vi "SpectrumCursor_getCenter.vi"(5 "Value":cluster{dbl[], dbl[]}) -> (0 "cursor2X":i64, 1 "cursor1X":i64)   [LabVIEW 2010]
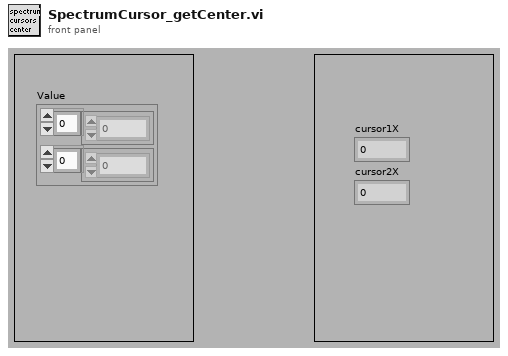
[diagram p1: front panel]
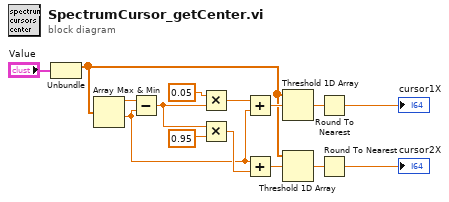
[diagram p0: block diagram]
diagram:
  n1 = Unbundle("Value") -> (w3:dbl[])  [unwired: 1 out]
  n2 = Array Max & Min(array=w3) -> (max value=w9:dbl, min value=w8:dbl)  [unwired: 2 out]
  n3 = Subtract(x=w9, y=w8) -> (x-y=w14:dbl)
  n4 = Multiply(x=0.05, y=w14) -> (x*y=w12:dbl)
  n5 = Multiply(x=w14, y=0.95) -> (x*y=w11:dbl)
  n6 = Add(x=w12, y=w8) -> (x+y=w7:dbl)
  n7 = Add(x=w8, y=w11) -> (x+y=w6:dbl)
  n8 = Threshold 1D Array(2:w7, 3:w3) -> (0:w4:dbl)  [unwired: 1 in]
  n9 = Threshold 1D Array(2:w6, 3:w3) -> (0:w5:dbl)  [unwired: 1 in]
  n10 = Round To Nearest(number=w4) -> (nearest integer value=→"cursor1X":dbl)
  n11 = Round To Nearest(number=w5) -> (nearest integer value=→"cursor2X":dbl)
